vi "1BS3HD_Scope_v00.vi"(0 "Scope+Safety":T1={"Safety First"={"lim reset"=FALSE, "no limit"=FALSE, "pos slew rate * dt"=12, "neg slew rate * dt"=-12, "Count(Ticks)"=0}, "Scope IPs"={"Trigger Direction"=enum."minus-plus", "Trigger Delay (ms)"=0.0, "Aquisition Rate (kHz)"=4000.0, "Trigger Offset (V)"=0.0, "Scale Offset"={"Scaling"={"Error signal"=1, "Output"=0, "DC Monitor"=1, "Threshold"=1}, "Offset"={"Error Signal"=0, "Output"=0, "DC Monitor"=0, "Threshold"=0}}}}, 9 "Scope":T2, 11 "Lock Select":T4, 12 "XY HD 3 ON":bool, 13 "XY HD 12 ON":bool, 14 "1SDI Data":u64[](array[numeric])) -> (1 "xy HD 1":cluster{i16[], i16[]}(graph), 2 "xy HD 2":cluster{i16[], i16[]}(graph), 3 "Scope OP 1SDI":cluster{dbl[], dbl[]}[](graph), 4 "xy HD 3":cluster{i16[], i16[]}(graph), 6 "Scope 1SDI ON":bool, 8 "error":dbl[](array[numeric]), 15 "Scope 1SDI FPGA":T3)   [LabVIEW 2013]
doc: "Creates an oscilliscope graph from the FIFO data, as well as packages data structures for FPGA_Cavities via the reference."
uses:
  Strict Type Defs/1BS3HD Lock Select.ctl
  Strict Type Defs/Lock or Hold.ctl
  Strict Type Defs/Scope and Safety.ctl
panel:
  out "Scope OPs (for saving)":cluster{dbl[], i16[], i16[], i16[], i16[]}
  in  "Scope":T3={"Trigger Direction"=enum."minus-plus", "Delay"=0, "Aquisition Rate (Ticks)"=20, "Offset"=0, "Channel"=0, "Channel Selector"={"Channel 1"=0, "Channel 2"=0, "Channel 3"=0, "Channel 4"=0}}
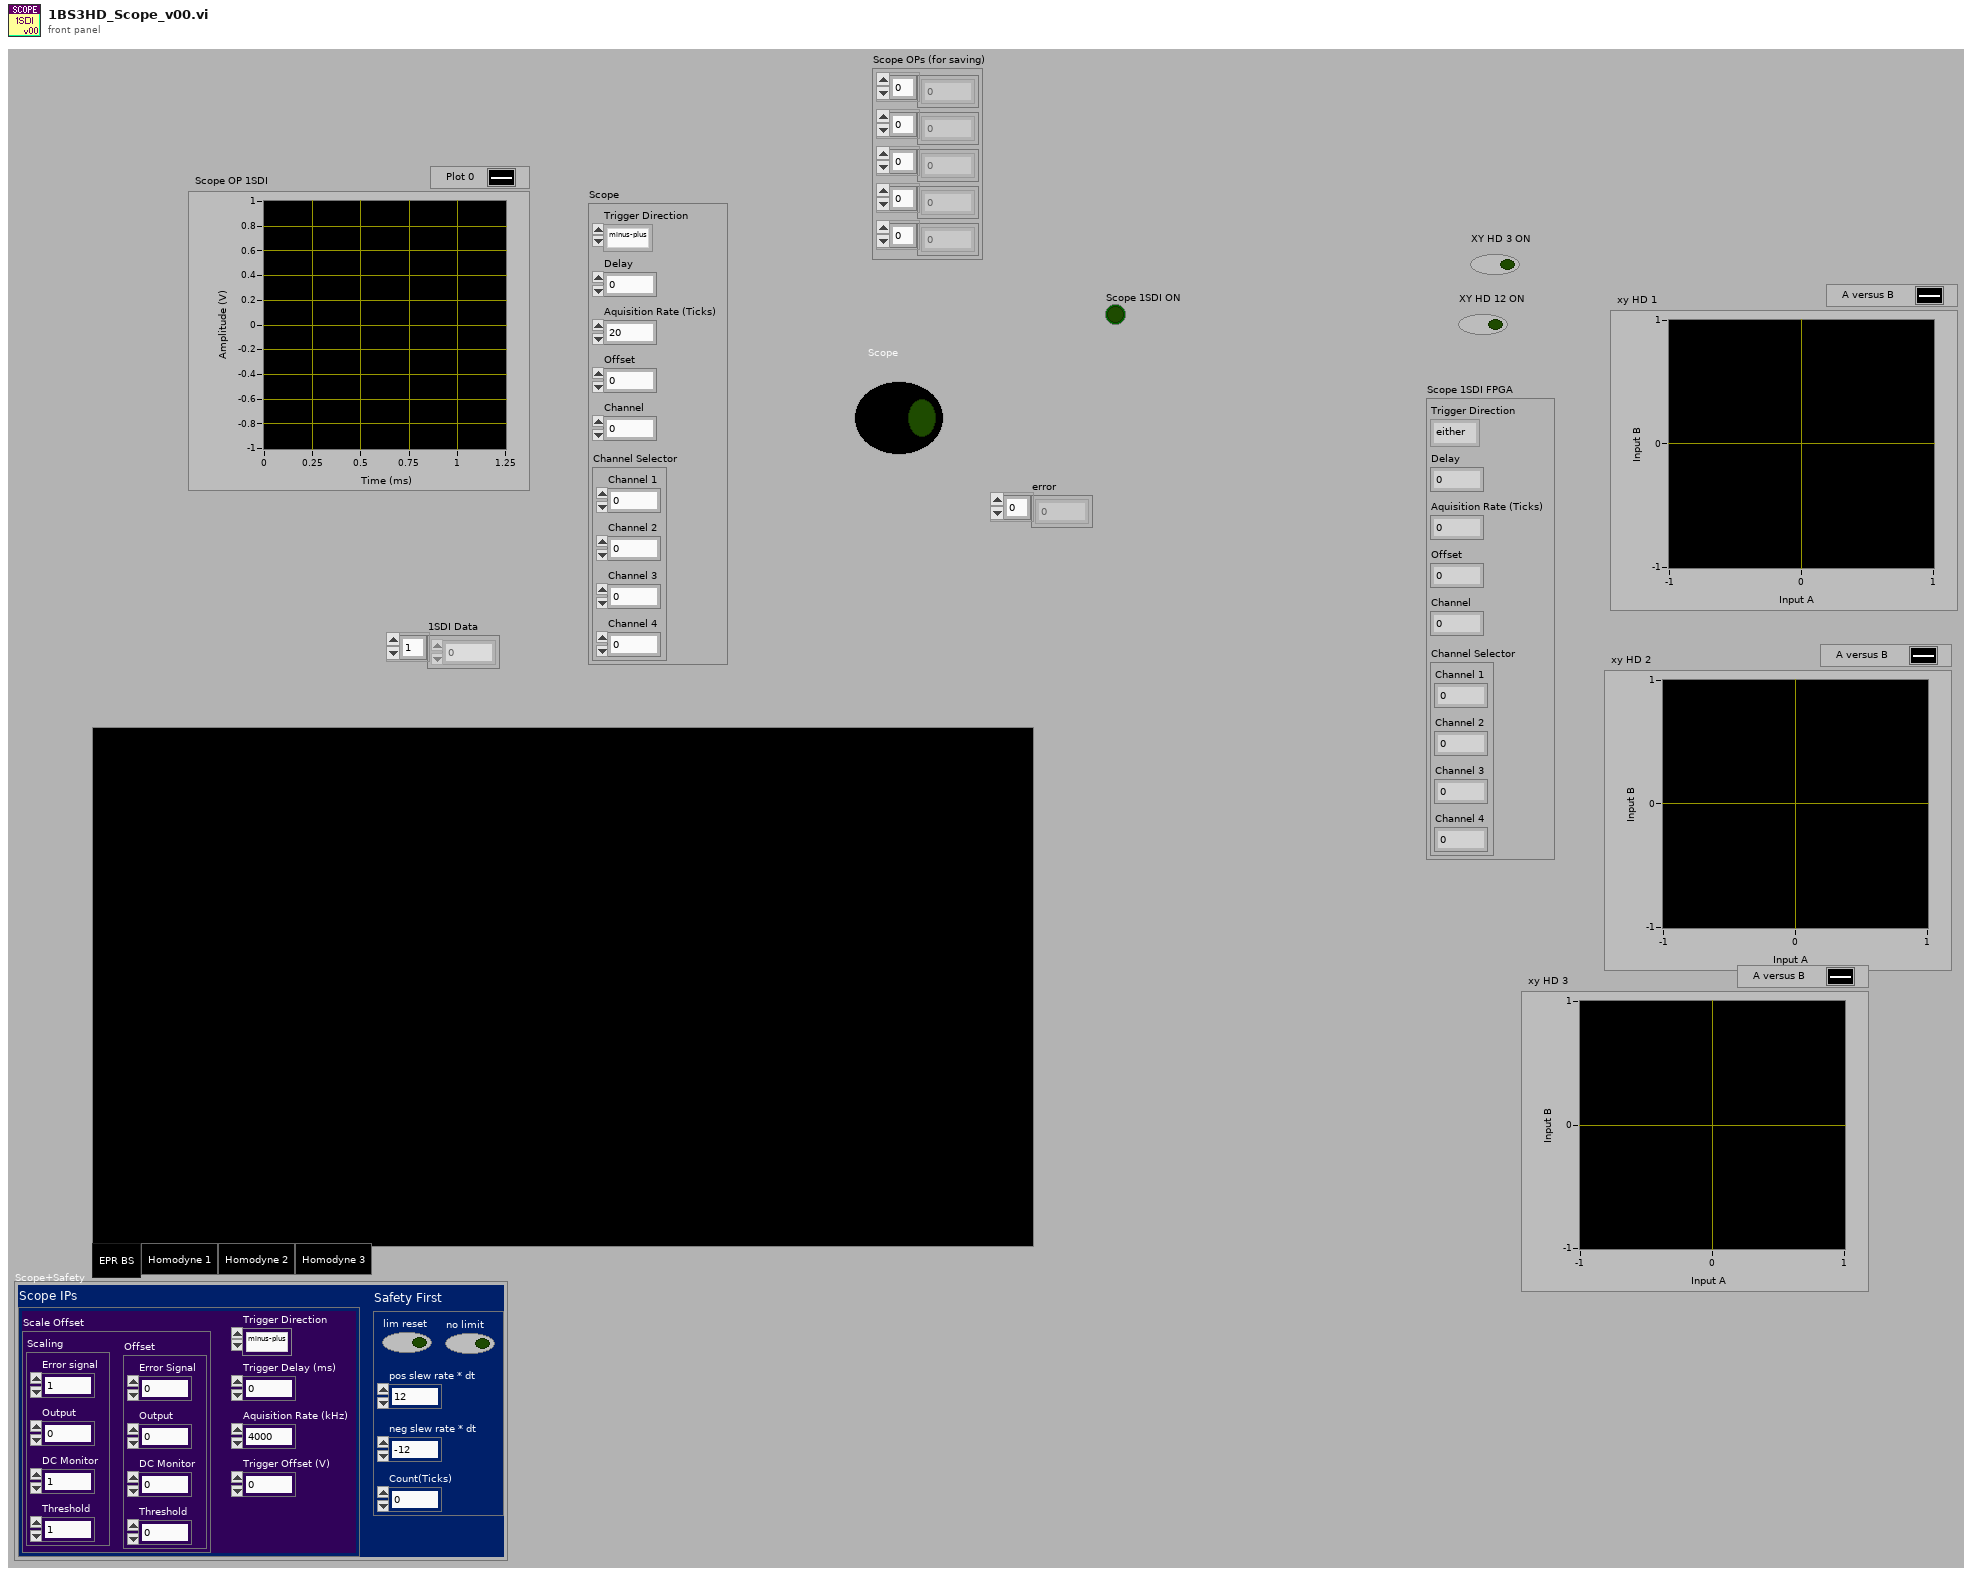
[diagram p1: front panel]
types:
  T1 = typedef "Scope and Safety.ctl" = cluster{"Safety First":cluster{"lim reset":bool, "no limit":bool, "pos slew rate * dt":i16, "neg slew rate * dt":i16, "Count(Ticks)":u32}, "Scope IPs":cluster{"Trigger Direction":enum8{"either", "minus-plus", "plus-minus"}, "Trigger Delay (ms)":dbl, "Aquisition Rate (kHz)":dbl, "Trigger Offset (V)":dbl, "Scale Offset":cluster{"Scaling":cluster{"Error signal":i16, "Output":i16, "DC Monitor":i16, "Threshold":i16}, "Offset":cluster{"Error Signal":i16, "Output":i16, "DC Monitor":i16, "Threshold":i16}}}}
  T2 = typedef "Lock or Hold.ctl" = bool
  T3 = cluster{"Trigger Direction":enum8{"either", "minus-plus", "plus-minus"}, "Delay":u32, "Aquisition Rate (Ticks)":u32, "Offset":i16, "Channel":i32, "Channel Selector":cluster{"Channel 1":i32, "Channel 2":i32, "Channel 3":i32, "Channel 4":i32}}
  T4 = typedef "1BS3HD Lock Select.ctl" = enum32{"EPR BS", "Homodyne 1", "Homodyne 2", "Homodyne 3"}
  T5 = cluster{"Channel 1":i32, "Channel 2":i32, "Channel 3":i32, "Channel 4":i32}
  T6 = cluster{"Trigger Direction":enum8{"either", "minus-plus", "plus-minus"}, "Trigger Delay (ms)":dbl, "Aquisition Rate (kHz)":dbl, "Trigger Offset (V)":dbl, "Scale Offset":cluster{"Scaling":cluster{"Error signal":i16, "Output":i16, "DC Monitor":i16, "Threshold":i16}, "Offset":cluster{"Error Signal":i16, "Output":i16, "DC Monitor":i16, "Threshold":i16}}}
  T7 = cluster{"Error signal":i16, "Output":i16, "DC Monitor":i16, "Threshold":i16}
  T8 = cluster{"Error Signal":i16, "Output":i16, "DC Monitor":i16, "Threshold":i16}
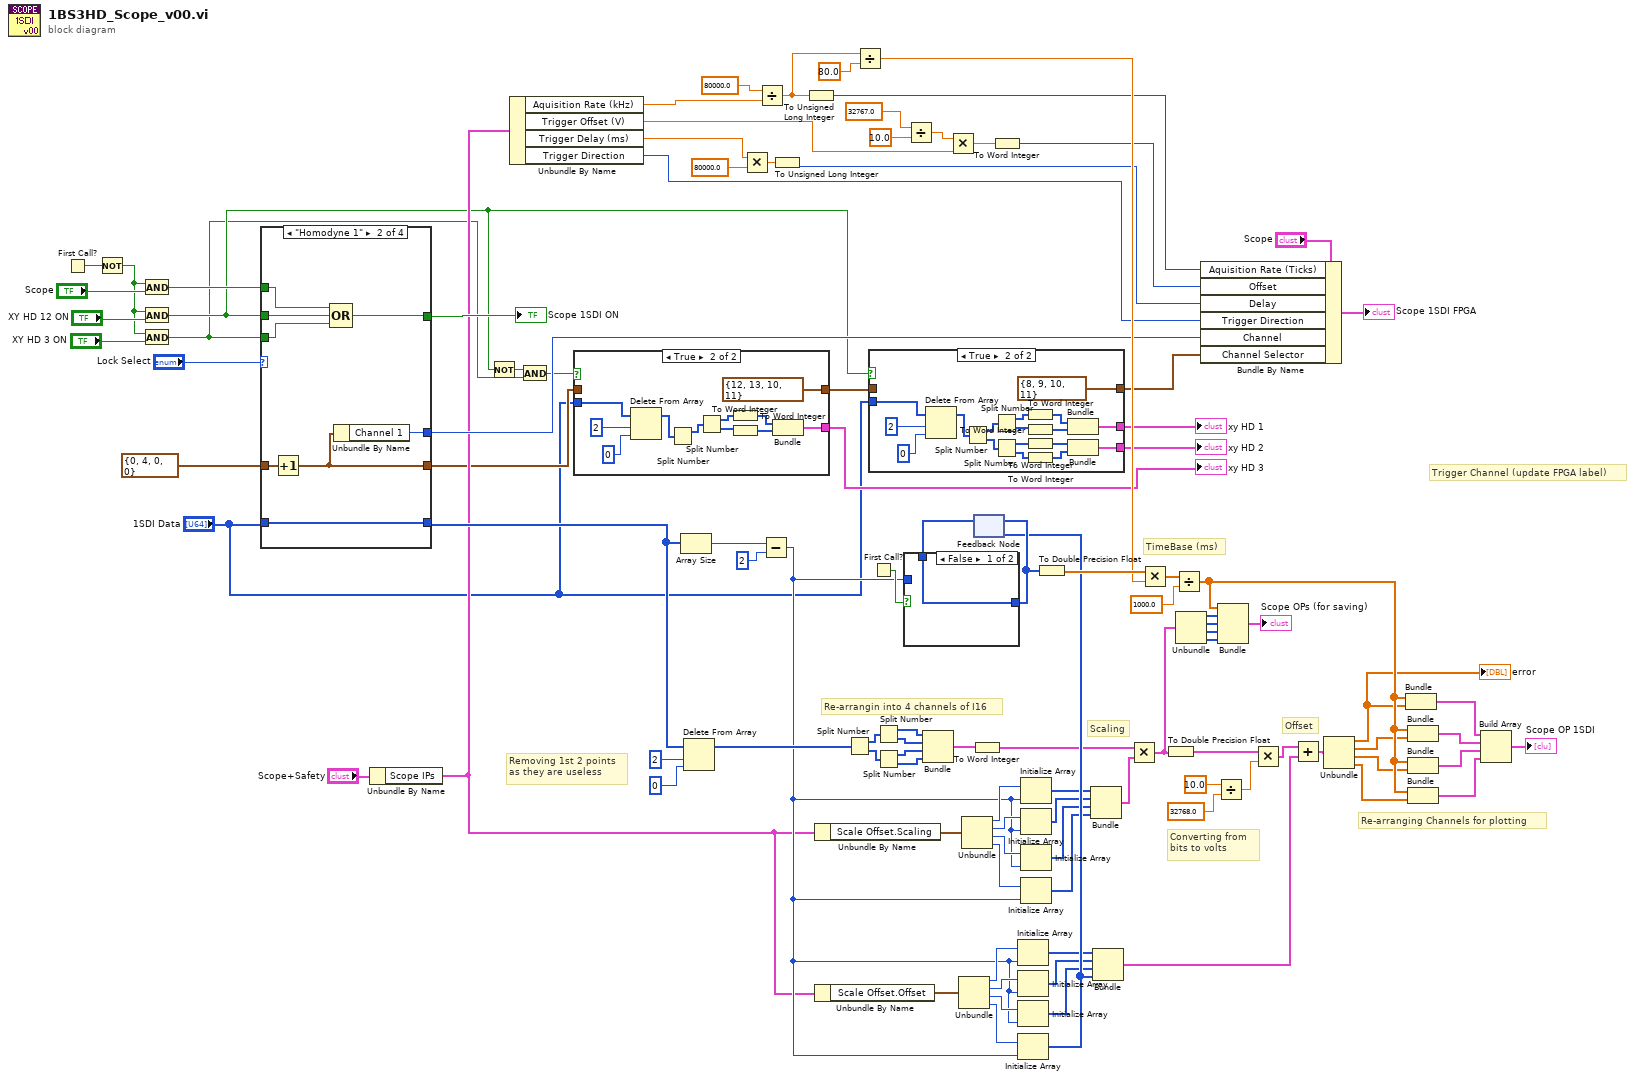
[diagram p0: block diagram]
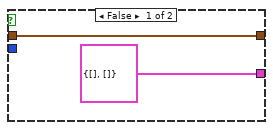
[diagram p2: hidden frame]
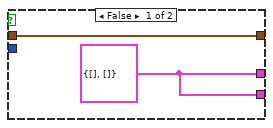
[diagram p3: hidden frame]
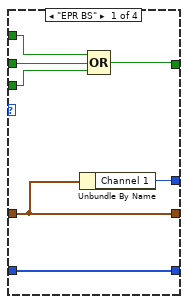
[diagram p5: hidden frame]
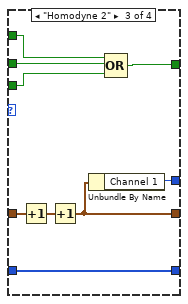
[diagram p6: hidden frame]
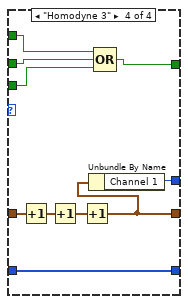
[diagram p7: hidden frame]
diagram:
  # "Trigger Channel (update FPGA label)"
  # "TimeBase (ms)"
  # "Re-arranging Channels for plotting"
  # "Re-arrangin into 4 channels of I16"
  # "Converting from\nbits to volts"
  # "Offset"
  # "Scaling"
  # "Removing 1st 2 points\nas they are useless"
  n1 = First Call?() -> (First Call?: T/F=w23:bool)
  n2 = Not(x=w23) -> (.not. x?=w9:bool)
  n3 = And(x=w9, y="Scope") -> (x .and. y?=w22:T2)
  n4 = And(x=w9, y="XY HD 12 ON") -> (x .and. y?=w2:bool)
  n5 = And(x=w9, y="XY HD 3 ON") -> (x .and. y?=w1:bool)
  n6 = case shown="\"Homodyne 1\"" "Lock Select" {
    tunnel: [w112 w119 w127 w137] -> w32
    tunnel: "1SDI Data" -> [w112 w119 w127 w137]
    tunnel: [w110 w118 w126 w136] -> w25
    tunnel: T5 {"Channel 1"=0, "Channel 2"=4, "Channel 3"=0, "Channel 4"=0} ("Channel Selector") -> [w111 w120 w129 w139]
    tunnel: [w111 w117 w125 w134] -> w7
    tunnel: w22 -> [w109 w116 w124 w133]
    tunnel: [w106 w113 w121 w130] -> w20
    tunnel: w2 -> [w108 w115 w123 w132]
    tunnel: w1 -> [w107 w114 w122 w131]
    frame "EPR BS" {
      n7 = Unbundle By Name(w111) -> ("Channel 1"=w110:i32)
      n8 = Compound Arithmetic op=OR(w109, w108, w107) -> (w106:T2)
    }
    frame "Homodyne 1" {
      n9 = Increment(x=w120) -> (x+1=w117:T5)
      n10 = Compound Arithmetic op=OR(w116, w115, w114) -> (w113:T2)
      n11 = Unbundle By Name(w117) -> ("Channel 1"=w118:i32)
    }
    frame "Homodyne 2" {
      n12 = Increment(x=w129) -> (x+1=w128:T5)
      n13 = Increment(x=w128) -> (x+1=w125:T5)
      n14 = Unbundle By Name(w125) -> ("Channel 1"=w126:i32)
      n15 = Compound Arithmetic op=OR(w124, w123, w122) -> (w121:T2)
    }
    frame "Homodyne 3" {
      n16 = Increment(x=w139) -> (x+1=w138:T5)
      n17 = Increment(x=w138) -> (x+1=w135:T5)
      n18 = Increment(x=w135) -> (x+1=w134:T5)
      n19 = Unbundle By Name(w134) -> ("Channel 1"=w136:i32)
      n20 = Compound Arithmetic op=OR(w133, w132, w131) -> (w130:T2)
    }
  }
  "Scope 1SDI ON" <- w20
  n21 = Unbundle By Name("Scope+Safety") -> ("Scope IPs"=w13:T6)
  n22 = Not(x=w2) -> (.not. x?=w4:bool)
  n23 = Unbundle By Name(w13) -> ("Aquisition Rate (kHz)"=w104:dbl, "Trigger Offset (V)"=w99:dbl, "Trigger Delay (ms)"=w97:dbl, "Trigger Direction"=w26:enum8{"either", "minus-plus", "plus-minus"})
  n24 = And(x=w4, y=w1) -> (x .and. y?=w3:bool)
  n25 = case shown="True" w3 {
    tunnel: w7 -> [w141 _]
    tunnel: [w141 T5 {"Channel 1"=12, "Channel 2"=13, "Channel 3"=10, "Channel 4"=11} ("Channel Selector")] -> w8
    tunnel: "1SDI Data" -> [_ w143]
    tunnel: [cluster{i16[], i16[]} {[], []} w146] -> w6
    frame False {
    }
    frame True {
      n26 = Delete From Array(array=w143, length=2, index=0) -> (array with subset deleted=w142:u64[])  [unwired: 1 out]
      n27 = Split Number(x=w142) -> (hi(x)=w150:u32[])  [unwired: 1 out]
      n28 = Split Number(x=w150) -> (hi(x)=w151:u16[], lo(x)=w149:u16[])
      n29 = To Word Integer(number=w151) -> (16bit integer=w148:i16[])
      n30 = To Word Integer(number=w149) -> (16bit integer=w147:i16[])
      n31 = Bundle(w148, w147) -> (w146:cluster{i16[], i16[]})  [unwired: 1 in]
    }
  }
  "xy HD 3" <- w6
  n32 = Array Size(array=w32) -> (size(s)=w90:i32)
  n33 = Delete From Array(array=w32, length=2, index=0) -> (array with subset deleted=w36:u64[])  [unwired: 1 out]
  n34 = Multiply(x=w97, y=80000.0) -> (x*y=w98:dbl)
  n35 = Divide(x=80000.0, y=w104) -> (x/y=w94:dbl)
  n36 = Subtract(x=w90, y=2) -> (x-y=w19:i32)
  n37 = To Unsigned Long Integer(number=w98) -> (unsigned 32bit integer=w27:u32)
  n38 = To Unsigned Long Integer(number=w94) -> (unsigned 32bit integer=w29:u32)
  n39 = Unbundle By Name(w13) -> ("Scale Offset.Scaling"=w61:T7)
  n40 = Unbundle By Name(w13) -> ("Scale Offset.Offset"=w45:T8)
  n41 = Split Number(x=w36) -> (hi(x)=w38:u32[], lo(x)=w37:u32[])
  n42 = Divide(x=w94, y=80.0) -> (x/y=w35:dbl)
  n43 = case shown="True" w2 {
    tunnel: w8 -> [w154 _]
    tunnel: [w154 T5 {"Channel 1"=8, "Channel 2"=9, "Channel 3"=10, "Channel 4"=11} ("Channel Selector")] -> w17
    tunnel: "1SDI Data" -> [_ w156]
    tunnel: [w153 w160] -> w16
    tunnel: [w153 w159] -> w15
    frame False {
      w153 = cluster{i16[], i16[]} {[], []}
    }
    frame True {
      n44 = Delete From Array(array=w156, length=2, index=0) -> (array with subset deleted=w155:u64[])  [unwired: 1 out]
      n45 = Split Number(x=w155) -> (hi(x)=w169:u32[], lo(x)=w165:u32[])
      n46 = Split Number(x=w169) -> (hi(x)=w170:u16[], lo(x)=w168:u16[])
      n47 = Split Number(x=w165) -> (hi(x)=w164:u16[], lo(x)=w163:u16[])
      n48 = To Word Integer(number=w170) -> (16bit integer=w167:i16[])
      n49 = To Word Integer(number=w168) -> (16bit integer=w166:i16[])
      n50 = To Word Integer(number=w164) -> (16bit integer=w161:i16[])
      n51 = To Word Integer(number=w163) -> (16bit integer=w162:i16[])
      n52 = Bundle(w167, w166) -> (w160:cluster{i16[], i16[]})  [unwired: 1 in]
      n53 = Bundle(w161, w162) -> (w159:cluster{i16[], i16[]})  [unwired: 1 in]
    }
  }
  "xy HD 1" <- w16
  "xy HD 2" <- w15
  n54 = First Call?() -> (First Call?: T/F=w64:bool)
  n55 = Split Number(x=w38) -> (hi(x)=w86:u16[], lo(x)=w87:u16[])
  n56 = Split Number(x=w37) -> (hi(x)=w88:u16[], lo(x)=w89:u16[])
  n57 = Divide(x=32767.0, y=10.0) -> (x/y=w102:dbl)
  n58 = Bundle(w86, w87, w88, w89) -> (w62:cluster{u16[], u16[], u16[], u16[]})  [unwired: 1 out]
  n59 = Multiply(x=w102, y=w99) -> (x*y=w103:dbl)
  n60 = Unbundle(w45) -> ("Error Signal"=w44:i16, "Output"=w48:i16, "DC Monitor"=w47:i16, "Threshold"=w46:i16)
  n61 = Unbundle(w61) -> ("Error signal"=w58:i16, "Output"=w57:i16, "DC Monitor"=w59:i16, "Threshold"=w60:i16)
  n62 = To Word Integer(number=w62) -> (16bit integer=w63:cluster{i16[], i16[], i16[], i16[]})
  n63 = To Word Integer(number=w103) -> (16bit integer=w28:i16)
  n64 = Initialize Array(w44, w19) -> (w49:i16[])
  n65 = Initialize Array(w48, w19) -> (w50:i16[])
  n66 = Initialize Array(w47, w19) -> (w51:i16[])
  n67 = Initialize Array(w46, w19) -> (w65:i16[])
  n68 = feedback #1(w65) -> (w66:i32[])
  n69 = case shown="False" w64 {
    tunnel: w19 -> [_ w174]
    tunnel: [w172 w173] -> w67
    tunnel: w66 -> [w172 _]
    frame False {
    }
    frame True {
      n70 = for {
        N: w174 -> [_]
        tunnel: [w175] -> w173 mode=indexing
        i -> [w175]
      }
    }
  }
  n71 = feedback-in #1(w67) -> ()
  n72 = Initialize Array(w58, w19) -> (w56:i16[])
  n73 = Initialize Array(w57, w19) -> (w55:i16[])
  n74 = Initialize Array(w59, w19) -> (w54:i16[])
  n75 = Initialize Array(w60, w19) -> (w53:i16[])
  n76 = To Double Precision Float(number=w67) -> (double precision float=w68:dbl[])
  n77 = Bundle(w56, w55, w54, w53) -> (w52:cluster{i16[], i16[], i16[], i16[]})  [unwired: 1 out]
  n78 = Bundle(w49, w50, w51, w65) -> (w43:cluster{i16[], i16[], i16[], i16[]})  [unwired: 1 out]
  n79 = Multiply(x=w63, y=w52) -> (x*y=w79:cluster{i16[], i16[], i16[], i16[]})
  n80 = Multiply(x=w68, y=w35) -> (x*y=w69:dbl[])
  n81 = To Double Precision Float(number=w79) -> (double precision float=w34:cluster{dbl[], dbl[], dbl[], dbl[]})
  n82 = Divide(x=w69, y=1000.0) -> (x/y=w84:dbl[])
  n83 = Unbundle(w79) -> (w80:i16[], w81:i16[], w82:i16[], w83:i16[])
  n84 = Bundle By Name(cluster="Scope", "Aquisition Rate (Ticks)"=w29, "Offset"=w28, "Delay"=w27, "Trigger Direction"=w26, "Channel"=w25, "Channel Selector"=w17) -> (→"Scope 1SDI FPGA":T3)
  n85 = Divide(x=10.0, y=32768.0) -> (x/y=w33:dbl)
  n86 = Bundle(w84, w80, w81, w82, w83) -> (→"Scope OPs (for saving)":cluster{dbl[], i16[], i16[], i16[], i16[]})  [unwired: 1 in]
  n87 = Multiply(x=w34, y=w33) -> (x*y=w41:cluster{dbl[], dbl[], dbl[], dbl[]})
  n88 = Add(x=w41, y=w43) -> (x+y=w42:cluster{dbl[], dbl[], dbl[], dbl[]})
  n89 = Unbundle(w42) -> (w11:dbl[], w71:dbl[], w72:dbl[], w73:dbl[])
  "error" <- w11
  n90 = Bundle(w84, w11) -> (w74:cluster{dbl[], dbl[]})  [unwired: 1 in]
  n91 = Bundle(w84, w71) -> (w75:cluster{dbl[], dbl[]})  [unwired: 1 in]
  n92 = Bundle(w84, w72) -> (w76:cluster{dbl[], dbl[]})  [unwired: 1 in]
  n93 = Bundle(w84, w73) -> (w77:cluster{dbl[], dbl[]})  [unwired: 1 in]
  n94 = Build Array(w74, w75, w76, w77) -> (→"Scope OP 1SDI":cluster{dbl[], dbl[]}[])
